vi "Initialize.vi"(8 "error in (no error)":errorcluster, 11 "Server in":refnum<class "Server.lvclass">) -> (0 "error out":errorcluster, 3 "Server out":refnum<class "Server.lvclass">)   [LabVIEW 2018, in "Server.lvclass"]
uses:
  Server.lvclass
  Server.lvclass/Server.ctl
  Comm/Stream/Stream.lvclass
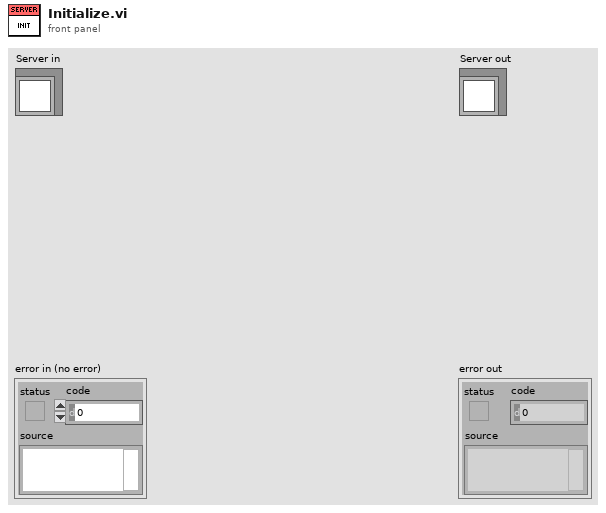
[diagram p1: front panel]
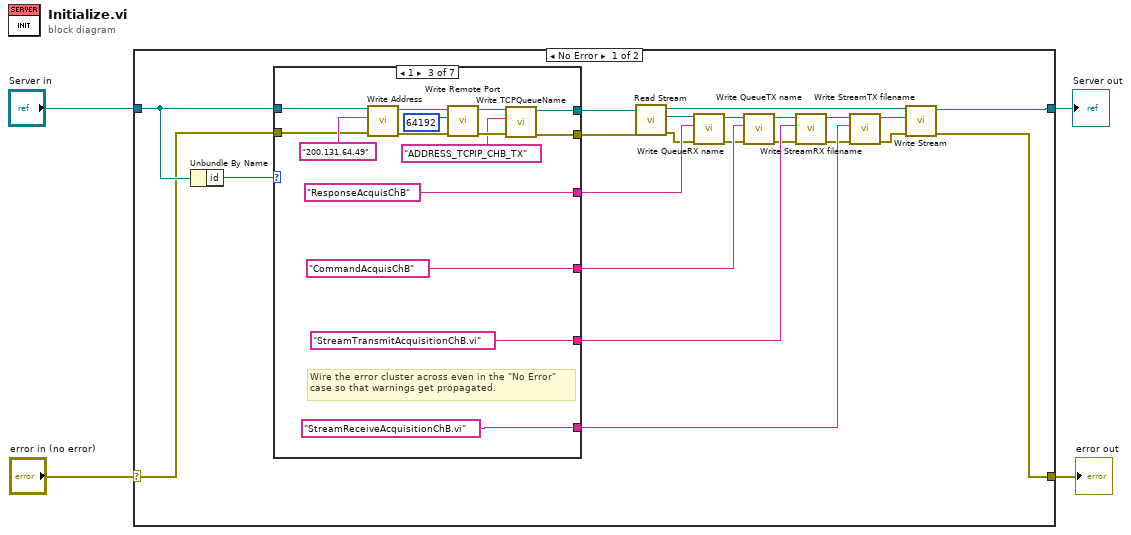
[diagram p0: block diagram]
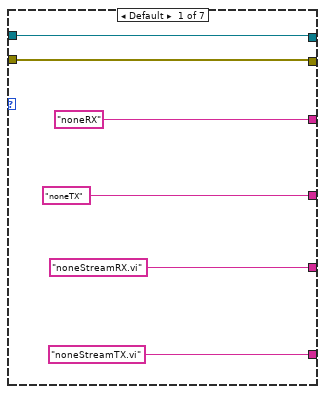
[diagram p2: hidden frame]
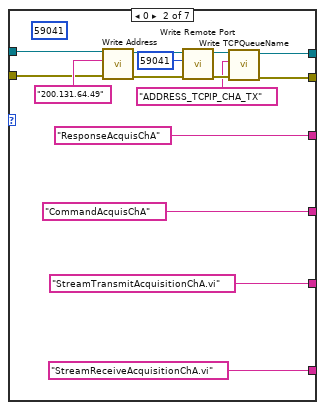
[diagram p3: hidden frame]
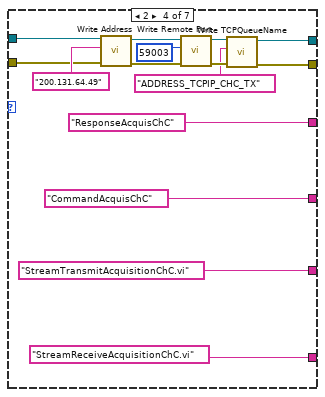
[diagram p4: hidden frame]
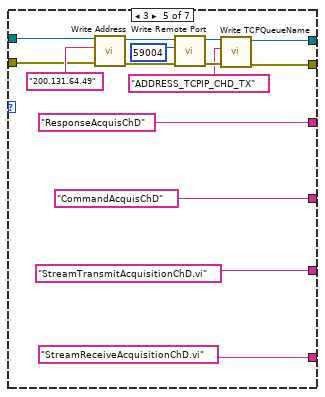
[diagram p5: hidden frame]
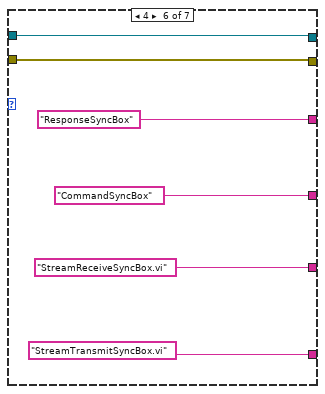
[diagram p6: hidden frame]
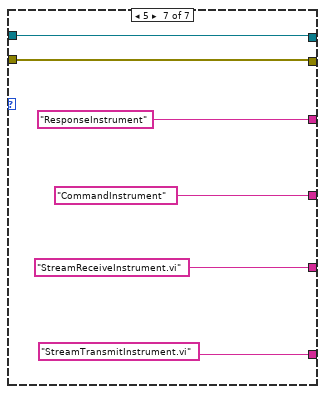
[diagram p7: hidden frame]
diagram:
  n1 = case shown="No Error" "error in (no error)" {
    selector: "error in (no error)" -> [w6 w106]
    tunnel: [w9 w106] -> w3
    tunnel: [w25 w105] -> w1
    tunnel: "Server in" -> [w8 w105]
    frame No Error {
      # "Wire the error cluster across even in the \"No Error\"\ncase so that warnings get propagated."
      n2 = Unbundle By Name(w8) -> ("id"=w24:u32)
      n3 = case shown="1" w24 {
        tunnel: ["noneRX" "ResponseAcquisChA" "ResponseAcquisChB" "ResponseAcquisChC" "ResponseAcquisChD" "ResponseSyncBox" "ResponseInstrument"] -> w23
        tunnel: ["noneStreamRX.vi" "StreamTransmitAcquisitionChA.vi" "StreamTransmitAcquisitionChB.vi" "StreamTransmitAcquisitionChC.vi" "StreamTransmitAcquisitionChD.vi" "StreamReceiveSyncBox.vi" "StreamReceiveInstrument.vi"] -> w16
        tunnel: ["noneStreamTX.vi" "StreamReceiveAcquisitionChA.vi" "StreamReceiveAcquisitionChB.vi" "StreamReceiveAcquisitionChC.vi" "StreamReceiveAcquisitionChD.vi" "StreamTransmitSyncBox.vi" "StreamTransmitInstrument.vi"] -> w15
        tunnel: ["noneTX" "CommandAcquisChA" "CommandAcquisChB" "CommandAcquisChC" "CommandAcquisChD" "CommandSyncBox" "CommandInstrument"] -> w22
        tunnel: w8 -> [w28 w37 w51 w66 w81 w94 w100]
        tunnel: [w28 w36 w49 w64 w78 w94 w100] -> w7
        tunnel: w6 -> [w27 w35 w50 w65 w80 w93 w99]
        tunnel: [w27 w34 w48 w63 w79 w93 w99] -> w5
        frame Default {
        }
        frame 0 {
          (unwired) u32 59041 ("Remote Port:")
          n4 = call "Write Address.vi"("error in (no error)"=w35, "Address"="200.131.64.49" ("Address:"), "Server in"=w37) -> ("error out"=w41:errorcluster, "Server out"=w40:refnum<class "Server.lvclass">)  [unwired: 7 in]
          n5 = call "Write Remote Port.vi"("error in (no error)"=w41, "Remote Port"=u32 59041, "Server in"=w40) -> ("error out"=w43:errorcluster, "Server out"=w42:refnum<class "Server.lvclass">)  [unwired: 7 in]
          n6 = call-dynamic "Write TCPQueueName.vi"("error in (no error)"=w43, "TCPQueueName"="ADDRESS_TCPIP_CHA_TX", "Server in"=w42) -> ("error out"=w34:errorcluster, "Server out"=w36:refnum<class "Server.lvclass">)  [unwired: 7 in]
        }
        frame 1 {
          n7 = call "Write Address.vi"("error in (no error)"=w50, "Address"="200.131.64.49" ("Address:"), "Server in"=w51) -> ("error out"=w56:errorcluster, "Server out"=w55:refnum<class "Server.lvclass">)  [unwired: 7 in]
          n8 = call "Write Remote Port.vi"("error in (no error)"=w56, "Remote Port"=u32 64192 ("Remote Port:"), "Server in"=w55) -> ("error out"=w58:errorcluster, "Server out"=w57:refnum<class "Server.lvclass">)  [unwired: 7 in]
          n9 = call-dynamic "Write TCPQueueName.vi"("error in (no error)"=w58, "TCPQueueName"="ADDRESS_TCPIP_CHB_TX", "Server in"=w57) -> ("error out"=w48:errorcluster, "Server out"=w49:refnum<class "Server.lvclass">)  [unwired: 7 in]
        }
        frame 2 {
          n10 = call "Write Address.vi"("error in (no error)"=w65, "Address"="200.131.64.49" ("Address:"), "Server in"=w66) -> ("error out"=w71:errorcluster, "Server out"=w70:refnum<class "Server.lvclass">)  [unwired: 7 in]
          n11 = call "Write Remote Port.vi"("error in (no error)"=w71, "Remote Port"=u32 59003 ("Remote Port:"), "Server in"=w70) -> ("error out"=w73:errorcluster, "Server out"=w72:refnum<class "Server.lvclass">)  [unwired: 7 in]
          n12 = call-dynamic "Write TCPQueueName.vi"("error in (no error)"=w73, "TCPQueueName"="ADDRESS_TCPIP_CHC_TX", "Server in"=w72) -> ("error out"=w63:errorcluster, "Server out"=w64:refnum<class "Server.lvclass">)  [unwired: 7 in]
        }
        frame 3 {
          n13 = call "Write Address.vi"("error in (no error)"=w80, "Address"="200.131.64.49" ("Address:"), "Server in"=w81) -> ("error out"=w86:errorcluster, "Server out"=w85:refnum<class "Server.lvclass">)  [unwired: 7 in]
          n14 = call "Write Remote Port.vi"("error in (no error)"=w86, "Remote Port"=u32 59004 ("Remote Port:"), "Server in"=w85) -> ("error out"=w88:errorcluster, "Server out"=w87:refnum<class "Server.lvclass">)  [unwired: 7 in]
          n15 = call-dynamic "Write TCPQueueName.vi"("error in (no error)"=w88, "TCPQueueName"="ADDRESS_TCPIP_CHD_TX", "Server in"=w87) -> ("error out"=w79:errorcluster, "Server out"=w78:refnum<class "Server.lvclass">)  [unwired: 7 in]
        }
        frame 4 {
        }
        frame 5 {
        }
      }
      n16 = call-dynamic "Read Stream.vi"("error in (no error)"=w5, "Server in"=w7) -> ("error out"=w14:errorcluster, "Stream.lvclass"=w21:refnum<class "Stream.lvclass">, "Server out"=w26:refnum<class "Server.lvclass">)  [unwired: 7 in]
      n17 = call-dynamic "Write QueueRX name.vi"("error in (no error)"=w14, "QueueRX name"=w23, "Stream in"=w21) -> ("error out"=w13:errorcluster, "Stream out"=w20:refnum<class "Stream.lvclass">)  [unwired: 7 in]
      n18 = call-dynamic "Write QueueTX name.vi"("error in (no error)"=w13, "QueueTX name"=w22, "Stream in"=w20) -> ("error out"=w12:errorcluster, "Stream out"=w19:refnum<class "Stream.lvclass">)  [unwired: 7 in]
      n19 = call-dynamic "Write StreamRX filename.vi"("error in (no error)"=w12, "StreamRX filename"=w16, "Stream in"=w19) -> ("error out"=w11:errorcluster, "Stream out"=w18:refnum<class "Stream.lvclass">)  [unwired: 7 in]
      n20 = call-dynamic "Write StreamTX filename.vi"("error in (no error)"=w11, "StreamTX filename"=w15, "Stream in"=w18) -> ("error out"=w10:errorcluster, "Stream out"=w17:refnum<class "Stream.lvclass">)  [unwired: 7 in]
      n21 = call-dynamic "Write Stream.vi"("error in (no error)"=w10, "Stream.lvclass"=w17, "Server in"=w26) -> ("error out"=w9:errorcluster, "Server out"=w25:refnum<class "Server.lvclass">)  [unwired: 7 in]
    }
    frame Error {
    }
  }
  "error out" <- w3
  "Server out" <- w1
